vi "Msg To.vi"() -> (3 "Setup Msg out":refnum<class "Setup Msg Strategy.lvclass">)   [LabVIEW 2021, in "jettl.lvlib" / "Setup.lvlib" / "Setup Msg Strategy.lvclass"]
uses:
  Setup Msg Strategy.lvclass
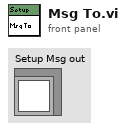
[diagram p1: front panel]
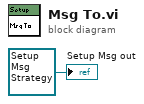
[diagram p0: block diagram]
diagram:
  "Setup Msg out" <- refnum<class "Setup Msg Strategy.lvclass"> refnum ("Setup Msg out")
